vi "Prototype.vi"(8 "error in (no error)":errorcluster, 11 "Abstract Message Rescripter in":refnum<class "Abstract Message Rescripter.lvclass">) -> (0 "error out":errorcluster, 3 "Abstract Message Rescripter out":refnum<class "Abstract Message Rescripter.lvclass">)   [LabVIEW 2020, in "Message Rescripter.lvlib" / "Abstract Message Rescripter.lvclass"]
uses:
  Abstract Message Rescripter.lvclass
  MessageMakerProvider/_Message Maker/_Maker Classes/Abstract Message Scripter/Abstract Message Scripter.lvclass
  MessageMakerProvider/_Message Maker/_Maker Classes/Message Scripter/Message Scripter.lvclass
  MessageMakerProvider/_Message Maker/Message Maker.lvlib
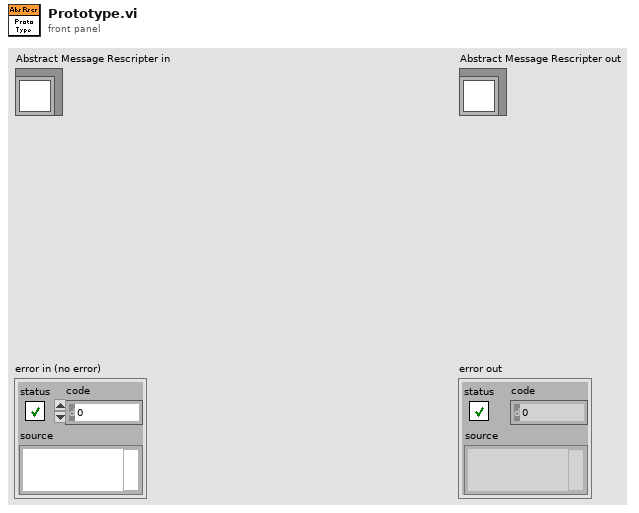
[diagram p1: front panel]
types:
  T1 = enum16{"Invalid Wire Rule", "Required", "Recommended", "Optional", "Dynamic Dispatch"}
  T2 = enum16{"Invalid Wire Rule", "Required", "Recommended", "Optional", "Dynamic Dispatch"}[]
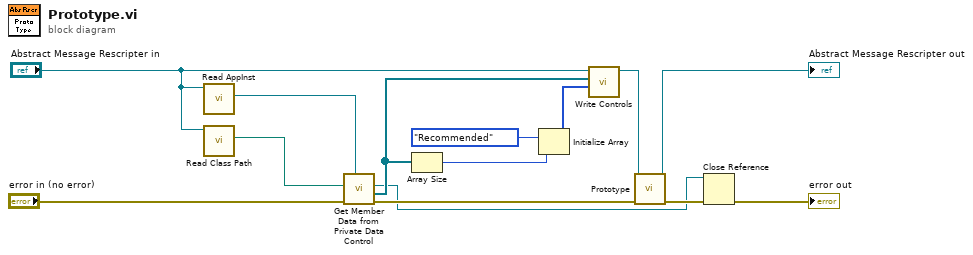
[diagram p0: block diagram]
diagram:
  n1 = call "Read AppInst.vi"("Message Maker in"="Abstract Message Rescripter in") -> ("AppInst"=w3:refnum<vi>)  [unwired: 10 in]
  n2 = call "Read Class Path.vi"("Message Scripter in"="Abstract Message Rescripter in") -> ("Class Path"=w1:path)  [unwired: 10 in]
  n3 = call "Get Member Data from Private Data Control.vi"("AppInst"=w3, "error in (no error)"="error in (no error)", "Target Path"=w1) -> ("error out"=w11:errorcluster, "Controls"=w8:refnum<vi>[], "Private data Control"=w4:refnum<vi>)  [unwired: 6 in]
  n4 = Array Size(array=w8) -> (size(s)=w9:i32)
  n5 = Initialize Array(T1."Recommended" ("Wire Rule"), w9) -> (w7:T2)
  n6 = call "Write Controls.vi"("Wiring Rules"=w7, "Controls[]"=w8, "Message Scripter in"="Abstract Message Rescripter in") -> ("Message Scripter out"=w13:refnum<class "Abstract Message Rescripter.lvclass">)  [unwired: 8 in]
  n7 = call-parent "Prototype.vi"("error in (no error)"=w11, "Message Scripter in"=w13) -> ("error out"=w14:errorcluster, "Message Scripter out"=→"Abstract Message Rescripter out":refnum<class "Abstract Message Rescripter.lvclass">)  [unwired: 8 in]
  n8 = Close Reference(reference=w4, error in (no error)=w14) -> (error out=→"error out":errorcluster)
